vi "Initialize OOB Communications.vi"(8 "error in (no error)":errorcluster, 11 "CIFTemplatePlugin in":refnum<class "TemplatePlugin.lvclass">) -> (0 "error out":errorcluster, 3 "CIFTemplatePlugin out":refnum<class "TemplatePlugin.lvclass">)   [LabVIEW 2021, in "TemplatePlugin.lvclass"]
uses:
  TemplatePlugin.lvclass
  TemplatePlugin.lvclass/TemplatePlugin.ctl
  OOB/OOB_Tx/TemplateOOB_Tx.lvclass
  OOB/OOB_Rx/TemplateOOB_Rx.lvclass
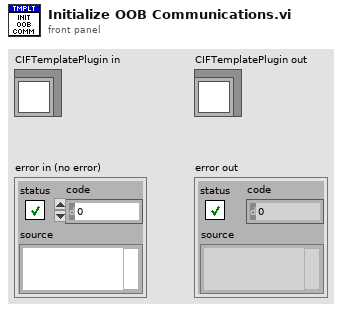
[diagram p1: front panel]
types:
  T1 = typedef "TemplatePlugin.lvclass/gRPC to Main Cyclic Data.ctl" = cluster{"Cyclic Data 1 -> Main":i32}
  T2 = typedef "TemplatePlugin.lvclass/Main to gRPC Cyclic Data.ctl" = cluster{" Cyclic Data 1 ->gRPC":i32}
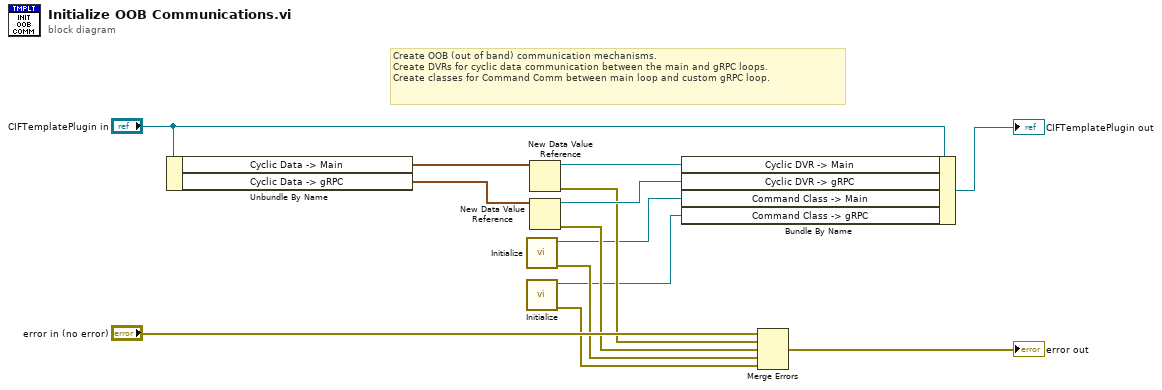
[diagram p0: block diagram]
diagram:
  # "Create OOB (out of band) communication mechanisms.\nCreate DVRs for cyclic data communication between the main and gRPC loops. \nCreate classes for Command Comm between main loop and custom gRPC loop."
  n1 = Unbundle By Name("CIFTemplatePlugin in") -> ("Cyclic Data -> Main"=w13:T1, "Cyclic Data -> gRPC"=w14:T2)
  n2 = call "Initialize.vi"() -> ("error out"=w4:errorcluster, "CutomOOB_Rx out"=w2:refnum<class "TemplateOOB_Rx.lvclass">)  [unwired: 10 in]
  n3 = call "Initialize.vi"() -> ("error out"=w3:errorcluster, "CutomOOB_Tx out"=w1:refnum<class "TemplateOOB_Tx.lvclass">)  [unwired: 10 in]
  n4 = New Data Value Reference(data value=w13) -> (data value reference=w10:refnum<data-value>, error out=w7:errorcluster)  [unwired: 1 in]
  n5 = New Data Value Reference(data value=w14) -> (data value reference=w9:refnum<data-value>, error out=w6:errorcluster)  [unwired: 1 in]
  n6 = Bundle By Name(cluster="CIFTemplatePlugin in", "Cyclic DVR -> Main"=w10, "Cyclic DVR -> gRPC"=w9, "Command Class -> Main"=w2, "Command Class -> gRPC"=w1) -> (→"CIFTemplatePlugin out":refnum<class "TemplatePlugin.lvclass">)
  n7 = Merge Errors("error in (no error)", w7, w6, w4, w3) -> (→"error out":errorcluster)
